vi "Query Max Channels.vi"(8 "error in (no error)":errorcluster, 11 "file path (dialog if empty)":path=path "/home/lvuser/Chad_Test.csv") -> (0 "error out":errorcluster, 2 "Num channels":string)   [LabVIEW 2019]
uses:
  <vilib>/Utility/file.llb/Read Delimited Spreadsheet (string).vi
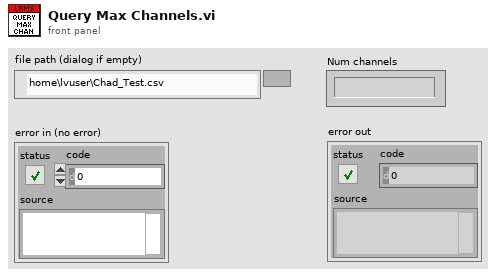
[diagram p1: front panel]
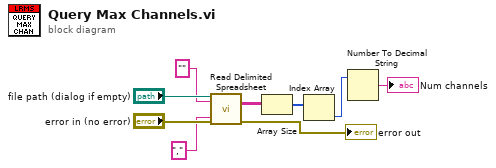
[diagram p0: block diagram]
diagram:
  n1 = call-poly <vilib>:"Read Delimited Spreadsheet.vi"("file path (dialog if empty)"="file path (dialog if empty)", "format (%s)"="" ("format (%.3f)"), "error in (no error)"="error in (no error)", "delimiter (\\t)"="," ("delimiter (\\t)")) -> ("all rows"=w5:string[][], "error out"=→"error out":errorcluster)  [unwired: 6 in, 4 out]
  n2 = Array Size(array=w5) -> (size(s)=w6:i32[])
  n3 = Index Array(array=w6) -> (element=w2:i32)  [unwired: 1 in]
  n4 = Number To Decimal String(number=w2) -> (decimal integer string=→"Num channels":string)  [unwired: 1 in]
